vi "Initialization.vi"(8 "error in (no error)":errorcluster caption="entrée d'erreur (pas d'erreur)", 10 "Container in":refnum<class "MDI Container.lvclass">, 11 "Container en entrée":refnum<class "Container.lvclass">) -> (0 "error out":errorcluster caption="sortie d'erreur", 2 "Container out":refnum<class "MDI Container.lvclass">, 3 "Container en sortie":refnum<class "Container.lvclass">)   [LabVIEW 2023, in "Container.lvclass"]
uses:
  Container.lvclass
  <vilib>/MGI/Panel Manager - .NET Panels/MDI/MDI Container/MDI Container.lvclass
  Container.lvclass/Container.ctl
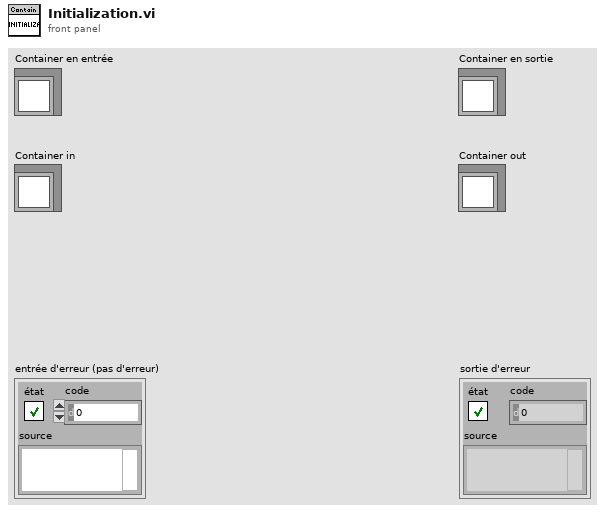
[diagram p1: front panel]
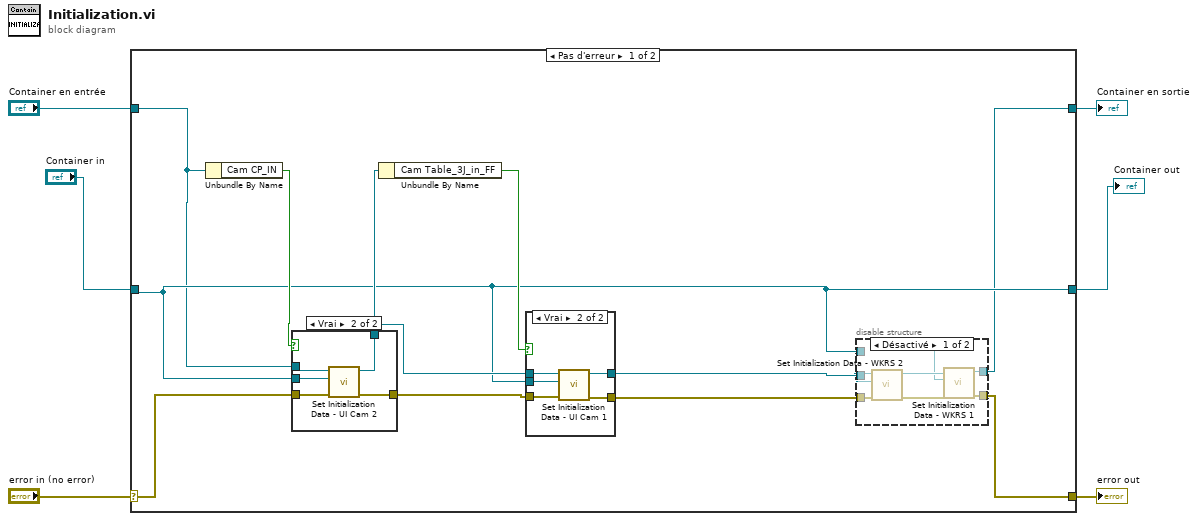
[diagram p0: block diagram]
diagram:
  n1 = case shown="Pas d'erreur" "error in (no error)" {
    selector: "error in (no error)" -> [w9 w43]
    tunnel: [w8 w43] -> w5
    tunnel: [w7 w42] -> w3
    tunnel: "Container en entrée" -> [w10 w42]
    tunnel: "Container in" -> [w11 w41]
    tunnel: [w11 w41] -> w1
    frame No Error {
      n2 = Unbundle By Name(w10) -> ("Cam CP_IN"=w13:bool)
      n3 = case shown="Vrai" w13 {
        tunnel: w9 -> [w18 w24]
        tunnel: [w18 w23] -> w15
        tunnel: w11 -> [_ w22]
        tunnel: w10 -> [w19 w21]
        tunnel: [w19 w20] -> w12
        frame False {
        }
        frame True {
          n4 = call "Set Initialization Data - UI Cam 2.vi"("error in"=w24, "Container"=w22, "Container in"=w21) -> ("error out"=w23:errorcluster, "Container out"=w20:refnum<class "Container.lvclass">)  [unwired: 7 in]
        }
      }
      n5 = Unbundle By Name(w12) -> ("Cam Table_3J_in_FF"=w14:bool)
      n6 = case shown="Vrai" w14 {
        tunnel: w15 -> [w25 w31]
        tunnel: [w25 w30] -> w17
        tunnel: [w26 w29] -> w16
        tunnel: w11 -> [_ w28]
        tunnel: w12 -> [w26 w27]
        frame False {
        }
        frame True {
          n7 = call "Set Initialization Data - UI Cam 1.vi"("error in"=w31, "Container"=w28, "Container in"=w27) -> ("error out"=w30:errorcluster, "Container out"=w29:refnum<class "Container.lvclass">)  [unwired: 7 in]
        }
      }
      n8 = disable-structure shown="Désactivé" {
        disable-tunnel: [w38 w39] -> w8
        disable-tunnel: [w37 w40] -> w7
        disable-tunnel: w17 -> [w34 w39]
        disable-tunnel: w16 -> [w33 w40]
        disable-tunnel: w11 -> [w32 _]
        frame Disabled {
          n9 = call "Set Initialization Data - WKRS 2.vi"("error in"=w34, "Container"=w32, "Container in"=w33) -> ("error out"=w36:errorcluster, "Container out"=w35:refnum<class "Container.lvclass">)  [unwired: 7 in]
          n10 = call "Set Initialization Data - WKRS 1.vi"("error in"=w36, "Container"=w32, "Container in"=w35) -> ("error out"=w38:errorcluster, "Container out"=w37:refnum<class "Container.lvclass">)  [unwired: 7 in]
        }
        frame Enabled {
        }
      }
    }
    frame Error {
    }
  }
  "error out" <- w5
  "Container en sortie" <- w3
  "Container out" <- w1
